vi "piezoTestCalibration.vi"() -> ()   [LabVIEW 2017]
uses:
  <vilib>/DAQmx/write.llb/DAQmx Write (Analog DBL 1Chan 1Samp).vi
  <vilib>/DAQmx/read.llb/DAQmx Read (Analog DBL 1Chan 1Samp).vi
  <vilib>/DAQmx/create/channels.llb/DAQmx Create Channel (AI-Voltage-Basic).vi
  <vilib>/DAQmx/miscellaneous.llb/DAQmx Fill In Error Info.vi
  <vilib>/DAQmx/create/channels.llb/DAQmx Create Channel (AO-Voltage-Basic).vi
  Piezo/lvlib/Madlib.lvlib
  <vilib>/Utility/file.llb/Write Delimited Spreadsheet (DBL).vi
panel:
  in  "piezo":i32
  out "read USB - set BNC vs set BNC":cluster{"X":dbl, "Y":dbl}[](graph)
  out "set vs desired":cluster{"X":dbl, "Y":dbl}[](graph)
  out "read USB - set USB vs set USB":cluster{"X":dbl, "Y":dbl}[](graph)
  out "read USB vs set USB":cluster{"X":dbl, "Y":dbl}[](graph)
  in  "N 2":i32
  out "read vs set (BNC)":cluster{"X":dbl, "Y":dbl}[](graph)
  out "expected-read vs set BNC":cluster{"X":dbl, "Y":dbl}[](graph)
  out "set USB - read BNC vs set USB":cluster{"X":dbl, "Y":dbl}[](graph)
  out "read BNC vs set USB":cluster{"X":dbl, "Y":dbl}[](graph)
  in  "N":i32
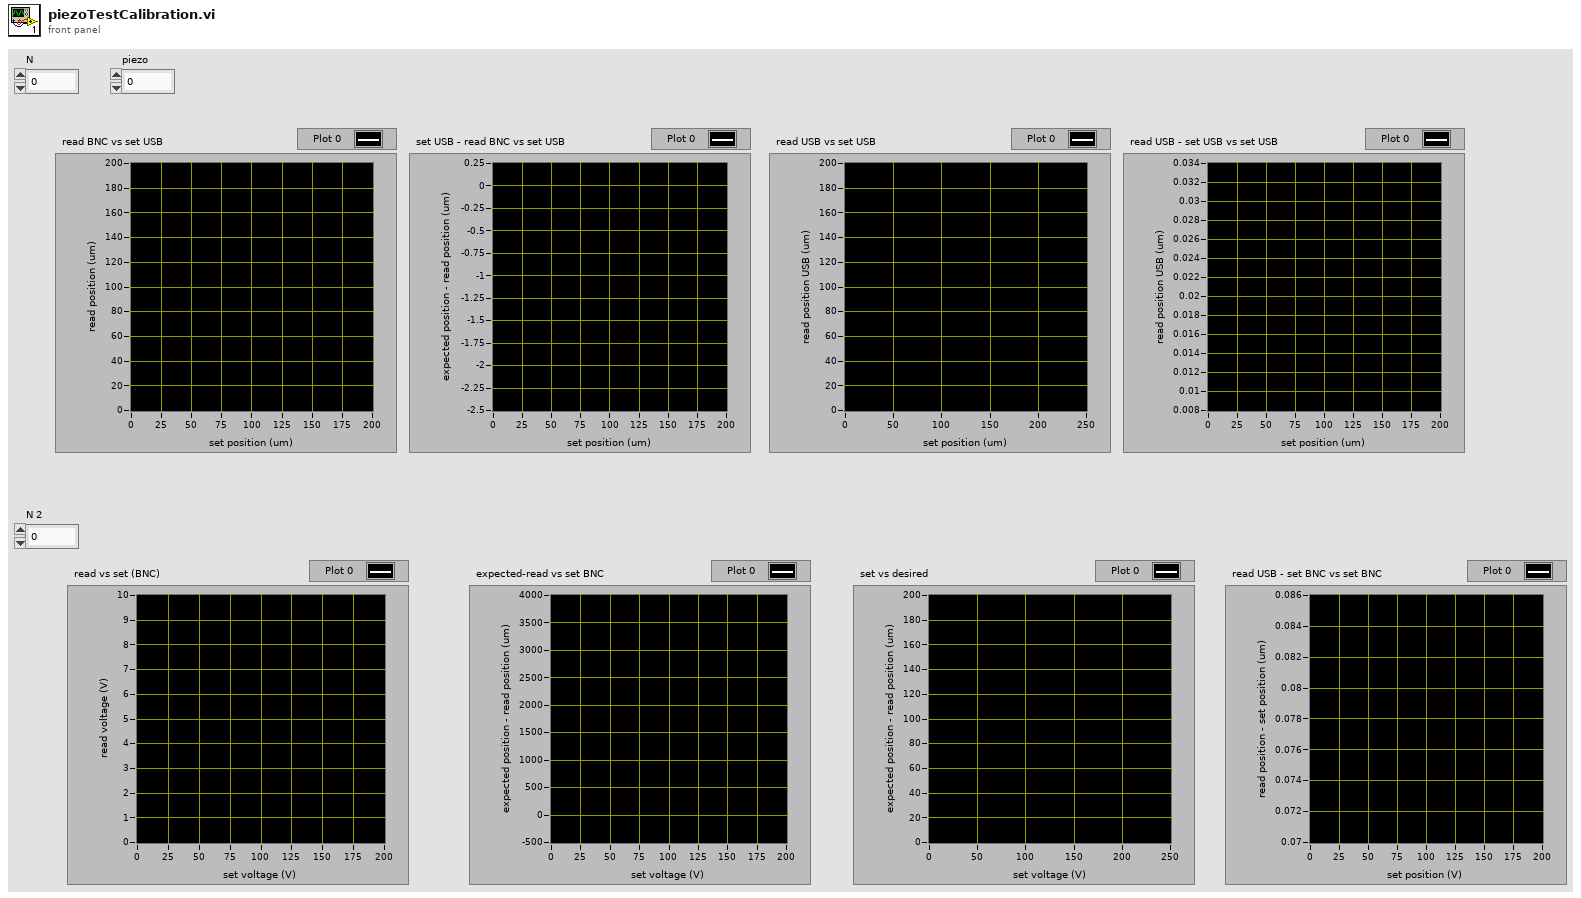
[diagram p1: front panel]
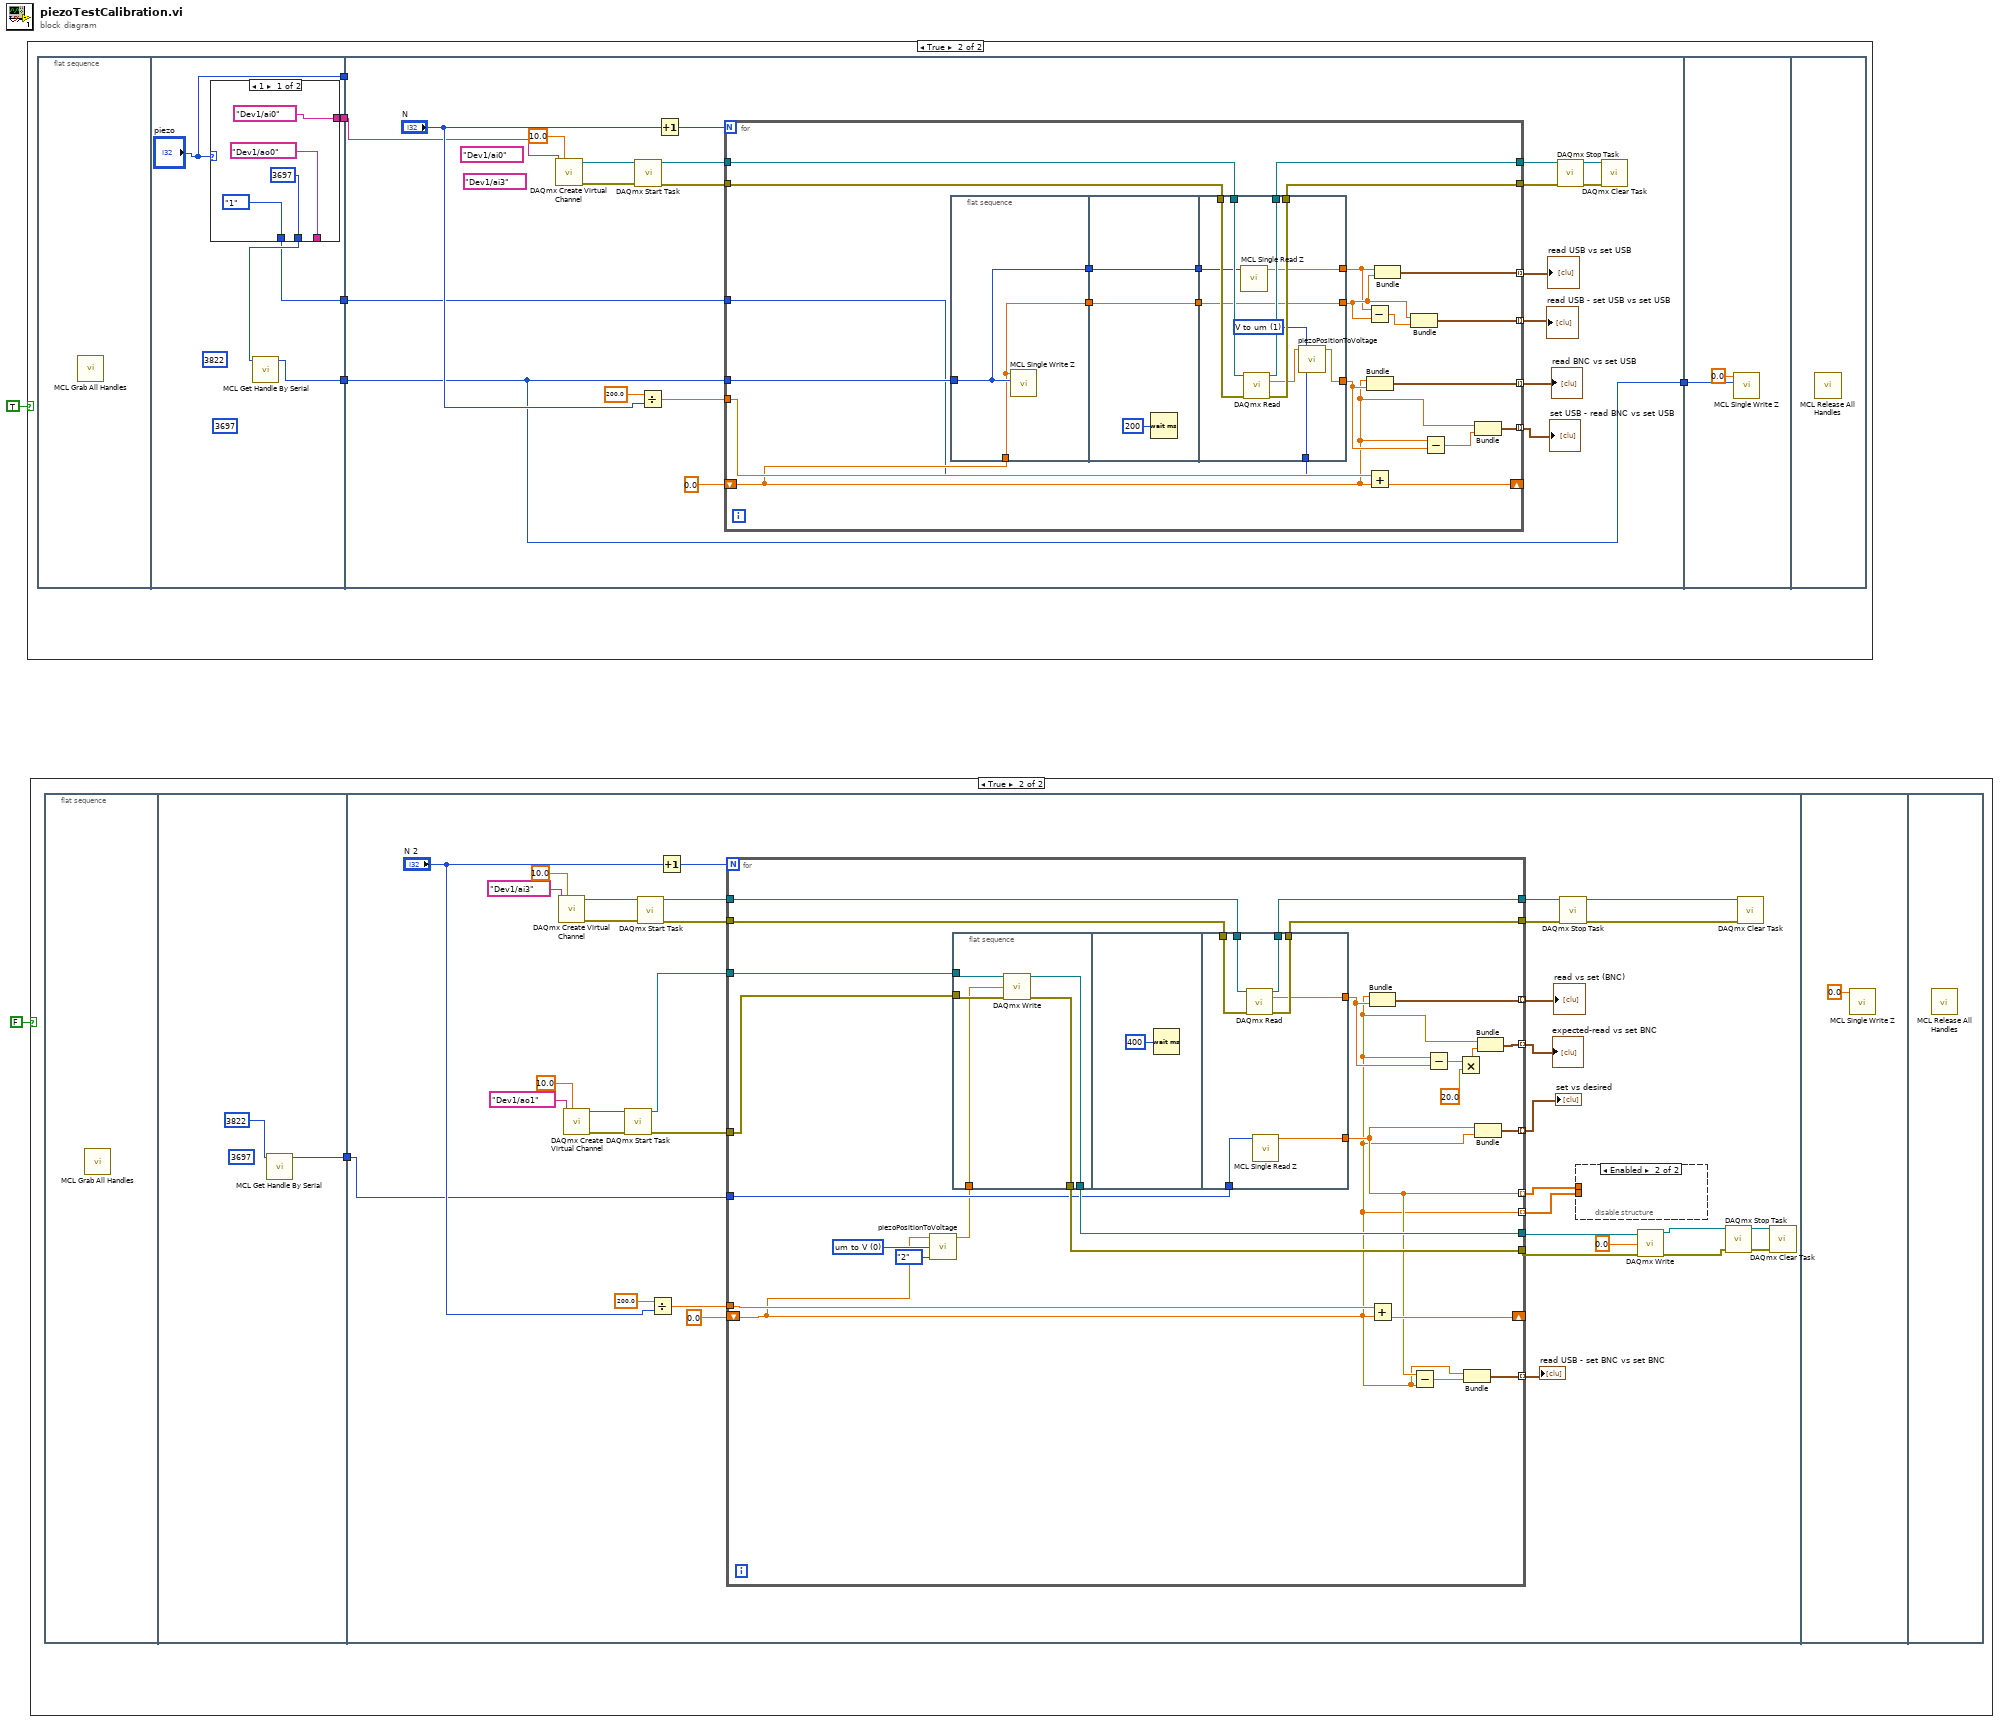
[diagram p0: block diagram]
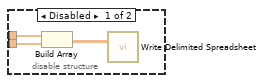
[diagram p3: hidden frame]
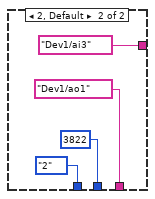
[diagram p5: hidden frame]
diagram:
  n1 = case shown="True" TRUE {
    frame False {
    }
    frame True {
      n2 = flat-sequence {
        tunnel: [w12] -> w7
        tunnel: [w10] -> w5
        tunnel: ["piezo"] -> w4
        tunnel: [w8] -> w3
        tunnel: w7 -> [w28]
        tunnel: [w28] -> w6
        tunnel: w5 -> [w22]
        tunnel: w4 -> [_]
        tunnel: w3 -> [w21]
        tunnel: w6 -> [w81]
        frame #0 {
          n3 = call "MCL Grab All Handles.vi"() -> ()  [unwired: 11 in, 1 out]
        }
        frame #1 {
          (unwired) i16 3697 ("serial")
          (unwired) i16 3822 ("serial")
          n4 = case shown="1" "piezo" {
            tunnel: [tag "Dev1/ai0" ("physical channels") tag "Dev1/ai3" ("physical channels")] -> w10
            tunnel: [tag "Dev1/ao0" ("physical channels") tag "Dev1/ao1" ("physical channels")] -> _
            tunnel: [i16 3697 ("serial") i16 3822 ("serial")] -> w11
            tunnel: [enum16{"1", "2"}."1" ("piezo") enum16{"1", "2"}."2" ("piezo")] -> w8
            frame 1 {
            }
            frame 2, Default {
            }
          }
          n5 = call "MCL Get Handle By Serial.vi"("serial"=w11) -> ("function return"=w12:i32)  [unwired: 10 in]
        }
        frame #2 {
          (unwired) tag "Dev1/ai3" ("physical channels")
          (unwired) tag "Dev1/ai0" ("physical channels")
          n6 = call-poly <vilib>:"DAQmx Create Virtual Channel.vi"("maximum value"=10.0, "physical channels"=w22) -> ("task out"=w41:refnum<k21>, "error out"=w40:errorcluster)  [unwired: 12 in]
          n7 = call <vilib>:"DAQmx Start Task.vi"("task/channels in"=w41, "error in"=w40) -> ("task out"=w39:refnum<k21>, "error out"=w38:errorcluster)  [unwired: 12 in]
          n8 = Divide(x=200.0, y="N") -> (x/y=w31:dbl)
          n9 = Increment(x="N") -> (x+1=w27:i32)
          n10 = for {
            N: w27 -> [_]
            tunnel: w39 -> [w63]
            tunnel: w38 -> [w62]
            tunnel: [w61] -> w37
            tunnel: [w60] -> w36
            tunnel: w31 -> [w59]
            shift-right: [w56] -> _
            shift-left: 0.0 -> [w44]
            tunnel: w28 -> [w58]
            tunnel: [w57] -> w26 mode=indexing
            tunnel: [w55] -> w25 mode=indexing
            tunnel: [w49] -> w24 mode=indexing
            tunnel: [w48] -> w23 mode=indexing
            tunnel: w21 -> [w42]
            n11 = flat-sequence {
              tunnel: w44 -> [w64]
              tunnel: w58 -> [w65]
              tunnel: [w65] -> w52
              tunnel: [w64] -> w50
              tunnel: [w67] -> w53
              tunnel: w52 -> [w67]
              tunnel: [w66] -> w51
              tunnel: w50 -> [w66]
              tunnel: w63 -> [w79]
              tunnel: w62 -> [w78]
              tunnel: [w77] -> w61
              tunnel: [w76] -> w60
              tunnel: [w70] -> w54
              tunnel: w53 -> [w75]
              tunnel: [w74] -> w45
              tunnel: [w73] -> w46
              tunnel: w51 -> [w73]
              tunnel: w42 -> [w69]
              frame #0 {
                n12 = call "MCL Single Write Z.vi"("handle"=w65, "position"=w64) -> ()  [unwired: 9 in, 1 out]
              }
              frame #1 {
                n13 = Wait (ms)(milliseconds to wait=u32 200) -> ()  [unwired: 1 out]
              }
              frame #2 {
                w72 = u16 1 items=["um to V", "V to um"] ("mode")
                n14 = call "MCL Single Read Z.vi"("handle"=w75) -> ("function return"=w74:dbl)  [unwired: 10 in]
                n15 = call-poly <vilib>:"DAQmx Read.vi"("task/channels in"=w79, "error in"=w78) -> ("task out"=w77:refnum<k21>, "data"=w71:dbl, "error out"=w76:errorcluster)  [unwired: 11 in]
                n16 = call "piezoPositionToVoltage.vi"("piezo"=w69, "mode"=w72, "in"=w71) -> ("out"=w70:dbl)  [unwired: 3 in, 1 out]
              }
            }
            n17 = Subtract(x=w45, y=w46) -> (x-y=w47:dbl)
            n18 = Bundle(w44, "out"=w54) -> (w57:cluster{dbl, "out":dbl})  [unwired: 1 in]
            n19 = Add(x=w59, y=w44) -> (x+y=w56:dbl)
            n20 = Bundle("function return"=w45, w46) -> (w49:cluster{"function return":dbl, dbl})  [unwired: 1 in]
            n21 = Bundle(w46, w47) -> (w48:cluster{dbl, dbl})  [unwired: 1 in]
            n22 = Subtract(x=w44, y=w54) -> (x-y=w43:dbl)
            n23 = Bundle(w44, w43) -> (w55:cluster{dbl, dbl})  [unwired: 1 in]
          }
          "read BNC vs set USB" <- w26
          "set USB - read BNC vs set USB" <- w25
          "read USB vs set USB" <- w24
          "read USB - set USB vs set USB" <- w23
          n24 = call <vilib>:"DAQmx Stop Task.vi"("task/channels in"=w37, "error in"=w36) -> ("task out"=w35:refnum<k21>, "error out"=w34:errorcluster)  [unwired: 12 in]
          n25 = call <vilib>:"DAQmx Clear Task.vi"("task in"=w35, "error in"=w34) -> ()  [unwired: 13 in, 1 out]
        }
        frame #3 {
          n26 = call "MCL Single Write Z.vi"("handle"=w81, "position"=0.0) -> ()  [unwired: 9 in, 1 out]
        }
        frame #4 {
          n27 = call "MCL Release All Handles.vi"() -> ()  [unwired: 12 in]
        }
      }
    }
  }
  n28 = case shown="True" FALSE {
    frame False {
    }
    frame True {
      n29 = flat-sequence {
        tunnel: [w84] -> w82
        tunnel: w82 -> [w89]
        frame #0 {
          n30 = call "MCL Grab All Handles.vi"() -> ()  [unwired: 11 in, 1 out]
        }
        frame #1 {
          (unwired) i16 3697 ("serial")
          n31 = call "MCL Get Handle By Serial.vi"("serial"=i16 3822) -> ("function return"=w84:i32)  [unwired: 10 in]
        }
        frame #2 {
          n32 = call-poly <vilib>:"DAQmx Create Virtual Channel.vi"("maximum value"=10.0, "physical channels"=tag "Dev1/ai3") -> ("task out"=w118:refnum<k21>, "error out"=w117:errorcluster)  [unwired: 12 in]
          n33 = call-poly <vilib>:"DAQmx Create Virtual Channel.vi"("maximum value"=10.0, "physical channels"=tag "Dev1/ao1") -> ("task out"=w100:refnum<k21>, "error out"=w99:errorcluster)  [unwired: 12 in]
          n34 = call <vilib>:"DAQmx Start Task.vi"("task/channels in"=w100, "error in"=w99) -> ("task out"=w98:refnum<k21>, "error out"=w97:errorcluster)  [unwired: 12 in]
          n35 = call <vilib>:"DAQmx Start Task.vi"("task/channels in"=w118, "error in"=w117) -> ("task out"=w116:refnum<k21>, "error out"=w115:errorcluster)  [unwired: 12 in]
          n36 = Divide(x=200.0, y="N 2") -> (x/y=w108:dbl)
          n37 = Increment(x="N 2") -> (x+1=w105:i32)
          n38 = for {
            N: w105 -> [_]
            tunnel: w116 -> [w147]
            tunnel: w115 -> [w146]
            tunnel: [w145] -> w114
            tunnel: [w144] -> w113
            tunnel: w108 -> [w143]
            shift-right: [w141] -> _
            shift-left: 0.0 -> [w124]
            tunnel: [w142] -> w104 mode=indexing
            tunnel: [w140] -> w103 mode=indexing
            tunnel: w98 -> [w135]
            tunnel: w97 -> [w134]
            tunnel: [w133] -> w94
            tunnel: [w132] -> w93
            tunnel: w89 -> [w131]
            tunnel: [w130] -> w88 mode=indexing
            tunnel: [w127] -> w87 mode=indexing
            tunnel: [w124] -> w86 mode=indexing
            tunnel: [w125] -> w85 mode=indexing
            w128 = u16 0 items=["um to V", "V to um"] ("mode")
            n39 = call "piezoPositionToVoltage.vi"("piezo"=enum16{"1", "2"}."2", "mode"=w128, "in"=w124) -> ("out"=w123:dbl)  [unwired: 3 in, 1 out]
            n40 = flat-sequence {
              tunnel: w123 -> [w148]
              tunnel: w135 -> [w152]
              tunnel: w134 -> [w151]
              tunnel: [w150] -> w133
              tunnel: [w149] -> w132
              tunnel: w147 -> [w160]
              tunnel: w146 -> [w159]
              tunnel: [w158] -> w145
              tunnel: [w157] -> w144
              tunnel: [w156] -> w138
              tunnel: w131 -> [w155]
              tunnel: [w154] -> w127
              frame #0 {
                n41 = call-poly <vilib>:"DAQmx Write.vi"("task/channels in"=w152, "data"=w148, "error in"=w151) -> ("task out"=w150:refnum<k21>, "error out"=w149:errorcluster)  [unwired: 10 in, 1 out]
              }
              frame #1 {
                n42 = Wait (ms)(milliseconds to wait=u32 400) -> ()  [unwired: 1 out]
              }
              frame #2 {
                n43 = call-poly <vilib>:"DAQmx Read.vi"("task/channels in"=w160, "error in"=w159) -> ("task out"=w158:refnum<k21>, "data"=w156:dbl, "error out"=w157:errorcluster)  [unwired: 11 in]
                n44 = call "MCL Single Read Z.vi"("handle"=w155) -> ("function return"=w154:dbl)  [unwired: 10 in]
              }
            }
            n45 = Bundle(w124, "data"=w138) -> (w142:cluster{dbl, "data":dbl})  [unwired: 1 in]
            n46 = Add(x=w143, y=w124) -> (x+y=w141:dbl)
            n47 = Subtract(x=w127, y=w124) -> (x-y=w126:dbl)
            n48 = Subtract(x=w124, y=w138) -> (x-y=w139:dbl)
            n49 = Multiply(x=w139, y=20.0) -> (x*y=w137:dbl)
            n50 = Bundle(w124, w126) -> (w125:cluster{dbl, dbl})  [unwired: 1 in]
            n51 = Bundle("function return"=w127, w124) -> (w130:cluster{"function return":dbl, dbl})  [unwired: 1 in]
            n52 = Bundle(w124, w137) -> (w140:cluster{dbl, dbl})  [unwired: 1 in]
          }
          "read vs set (BNC)" <- w104
          "expected-read vs set BNC" <- w103
          "set vs desired" <- w88
          "read USB - set BNC vs set BNC" <- w85
          n53 = call <vilib>:"DAQmx Stop Task.vi"("task/channels in"=w114, "error in"=w113) -> ("task out"=w112:refnum<k21>, "error out"=w111:errorcluster)  [unwired: 12 in]
          n54 = disable-structure shown="Enabled" {
            disable-tunnel: w87 -> [w122 _]
            disable-tunnel: w86 -> [w121 _]
            frame Disabled {
              n55 = Build Array(w122, w121) -> (w120:dbl[][])
              n56 = call-poly <vilib>:"Write Delimited Spreadsheet.vi"("2D data"=w120) -> ()  [unwired: 13 in, 2 out]
            }
            frame Enabled {
            }
          }
          n57 = call-poly <vilib>:"DAQmx Write.vi"("task/channels in"=w94, "data"=0.0, "error in"=w93) -> ("task out"=w92:refnum<k21>, "error out"=w91:errorcluster)  [unwired: 10 in, 1 out]
          n58 = call <vilib>:"DAQmx Stop Task.vi"("task/channels in"=w92, "error in"=w91) -> ("task out"=w95:refnum<k21>, "error out"=w96:errorcluster)  [unwired: 12 in]
          n59 = call <vilib>:"DAQmx Clear Task.vi"("task in"=w112, "error in"=w111) -> ()  [unwired: 13 in, 1 out]
          n60 = call <vilib>:"DAQmx Clear Task.vi"("task in"=w95, "error in"=w96) -> ()  [unwired: 13 in, 1 out]
        }
        frame #3 {
          n61 = call "MCL Single Write Z.vi"("position"=0.0) -> ()  [unwired: 10 in, 1 out]
        }
        frame #4 {
          n62 = call "MCL Release All Handles.vi"() -> ()  [unwired: 12 in]
        }
      }
    }
  }
